vi "initiate.vi"(8 "error in":errorcluster, 11 "Sub Panel":refnum<vi>) -> (0 "error out":errorcluster, 3 "simple_html_chat_ui out":refnum<class "simple_html_chat_ui.lvclass">)   [LabVIEW 2020, in "simple_html_chat_ui.lvclass"]
uses:
  simple_html_chat_ui.lvclass
  simple_html_chat_ui.lvclass/simple_html_chat_ui.ctl
  models/abstract_message_base/abstract_message_base.lvclass
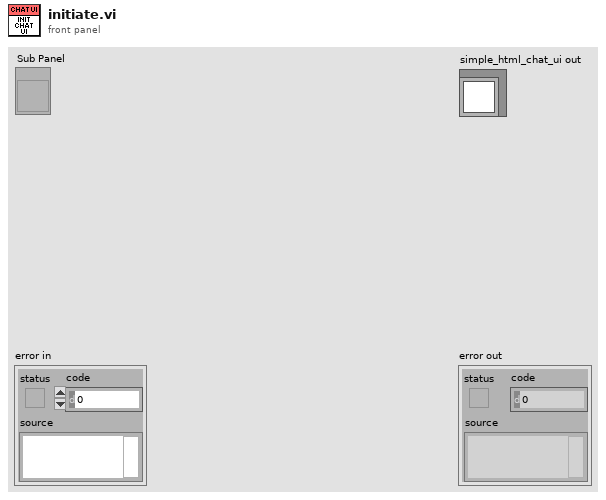
[diagram p1: front panel]
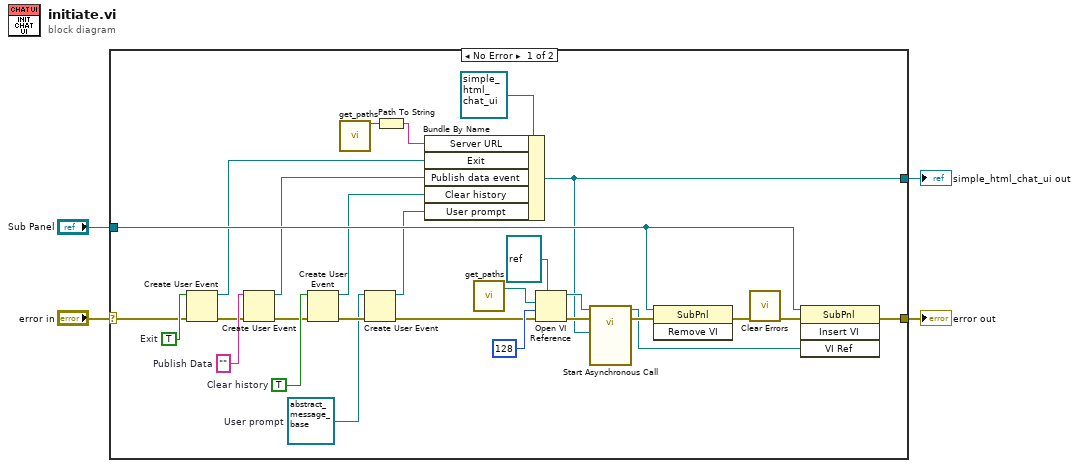
[diagram p0: block diagram]
diagram:
  n1 = case shown="No Error" "error in" {
    selector: "error in" -> [w20 w33]
    tunnel: [w30 w33] -> w4
    tunnel: [w12 _] -> w2
    tunnel: "Sub Panel" -> [w23 _]
    frame No Error {
      w5 = refnum<class "abstract_message_base.lvclass"> refnum  # User prompt
      w10 = TRUE  # Clear history
      w17 = ""  # Publish Data
      w21 = TRUE  # Exit
      n2 = Create User Event(user event datatype=w21, error in=w20) -> (user event=w18:refnum<user-event>, error out=w16:errorcluster)
      n3 = Create User Event(user event datatype=w17, error in=w16) -> (user event=w15:refnum<user-event>, error out=w7:errorcluster)
      n4 = Create User Event(user event datatype=w10, error in=w7) -> (user event=w9:refnum<user-event>, error out=w11:errorcluster)
      n5 = call "get_paths.vi"() -> ("html path"=w14:path)  [unwired: 18 in, 1 out]
      n6 = Create User Event(user event datatype=w5, error in=w11) -> (user event=w8:refnum<user-event>, error out=w6:errorcluster)
      n7 = Path To String(path=w14) -> (string=w13:string)
      n8 = Bundle By Name(cluster=refnum<class "simple_html_chat_ui.lvclass"> refnum ("simple_html_chat_ui in"), "Server URL"=w13, "Exit"=w18, "Publish data event"=w15, "Clear history"=w9, "User prompt"=w8) -> (w12:refnum<class "simple_html_chat_ui.lvclass">)
      n9 = call "get_paths.vi"() -> ("LV web ui path"=w22:path)  [unwired: 18 in, 1 out]
      n10 = Open VI Reference(type specifier VI Refnum (for type only)=refnum<vi> refnum, vi path=w22, options=128, error in (no error)=w6) -> (vi reference=w25:refnum<vi>, error out=w27:errorcluster)  [unwired: 2 in]
      n11 = call-by-ref "Start Asynchronous Call"(reference=w25, error in=w27, "simple_html_chat_ui in"=w12) -> (reference out=w24:refnum<vi>, error out=w26:errorcluster)  [unwired: 11 in]
      n12 = invoke class="SubPnl" method="Remove VI"(reference=w23, error in=w26) -> (error out=w32:errorcluster)  [unwired: 1 in, 2 out]
      n13 = call <vilib>:"Clear Errors.vi"("error in (no error)"=w32) -> ("error out"=w31:errorcluster)  [unwired: 5 in, 1 out]
      n14 = invoke class="SubPnl" method="Insert VI"(reference=w23, error in=w31, "VI Ref"=w24) -> (error out=w30:errorcluster)  [unwired: 1 in, 3 out]
    }
    frame Error {
    }
  }
  "error out" <- w4
  "simple_html_chat_ui out" <- w2
